vi "Test API Creates Report If No Tests Are Run.vi"(8 "error in (no error)":errorcluster, 11 "API Test in":refnum<class "API Test.lvclass">) -> (0 "error out":errorcluster, 3 "API Test out":refnum<class "API Test.lvclass">)   [LabVIEW 2020, in "LUnit Tests.lvlib" / "API Test.lvclass"]
uses:
  API Test.lvclass
  C:/Program Files (x86)/National Instruments/LabVIEW 2020/vi.lib/Astemes/LUnit/Test Case.lvclass
  <vilib>/Astemes/LUnit/Test Case.lvclass/Test Case.ctl
  <vilib>/Astemes/LUnit/Palette/Fail.vi
  <vilib>/Astemes/LUnit/Palette/Pass.vi
  <vilib>/Astemes/LUnit/Set Assertion Type.vi
  <vilib>/Astemes/LUnit/Add test result.vi
  <vilib>/Astemes/LUnit/LUnit Record Assertion Result.vi
  <vilib>/Astemes/LUnit/LUnit Aggregate Assertion Results.vi
  <vilib>/Astemes/LUnit/Method Result/LUnit Merge Status.vi
  <vilib>/Astemes/LUnit/LUnit Concatenate result strings.vi
  API Test.lvclass/API Test.ctl
  source/Framework/Execution API/Execution API.lvclass
  <vilib>/Astemes/LUnit/Test Case.lvclass
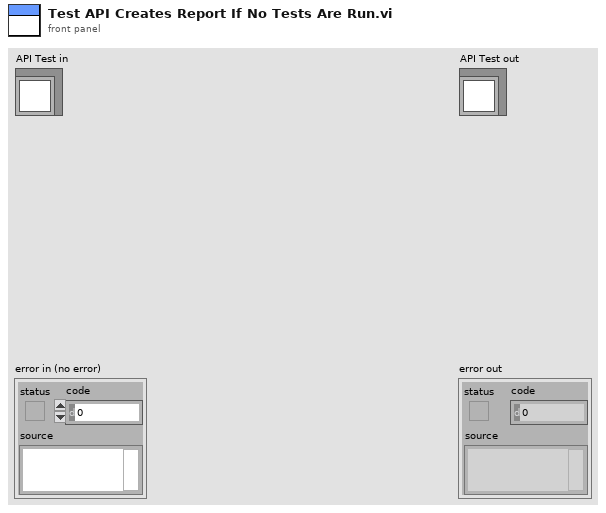
[diagram p1: front panel]
types:
  T1 = cluster{"Result Events":refnum<event-registration>, "Event Registration Refnum":refnum<event-registration>}
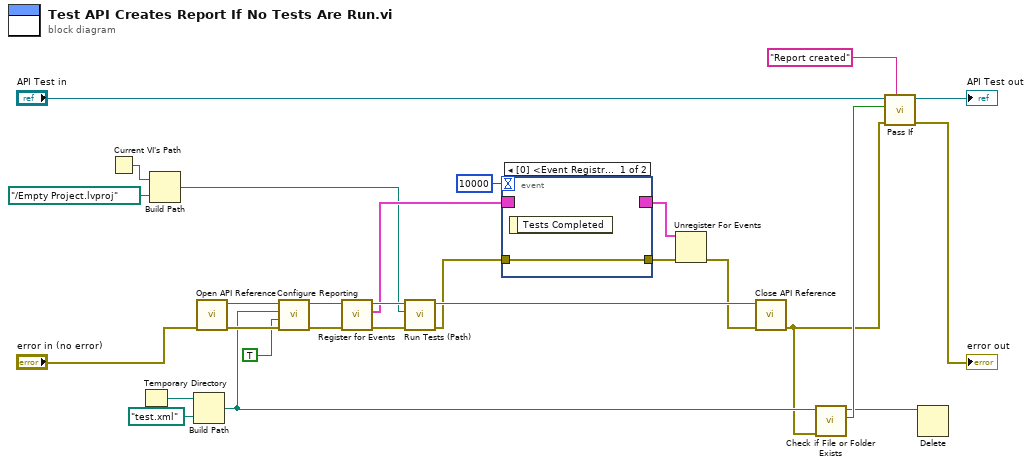
[diagram p0: block diagram]
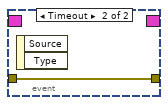
[diagram p2: hidden frame]
diagram:
  n1 = Current VI's Path() -> (path=w3:path)
  n2 = Temporary Directory() -> (w19:path)
  n3 = Build Path(base path=w3, name or relative path=path "../Empty Project.lvproj") -> (appended path=w1:path)
  n4 = Build Path(base path=w19, name or relative path=path "test.xml") -> (appended path=w16:path)
  n5 = call "Open API Reference.vi"("error in (no error)"="error in (no error)") -> ("error out"=w21:errorcluster, "Execution API out"=w22:refnum<class "Execution API.lvclass">)  [unwired: 9 in]
  n6 = call "Configure Reporting.vi"("error in (no error)"=w21, "Autogenerate?"=TRUE, "Path"=w16, "Execution API In"=w22) -> ("error out"=w20:errorcluster, "Execution API Out"=w6:refnum<class "Execution API.lvclass">)  [unwired: 6 in]
  n7 = call "Register for Events.vi"("error in (no error)"=w20, "Execution API in"=w6) -> ("error out"=w7:errorcluster, "Event Registrations"=w4:T1, "Execution API out"=w5:refnum<class "Execution API.lvclass">)  [unwired: 7 in]
  n8 = call "Run Tests (Path).vi"("error in (no error)"=w7, "Project or Class Path"=w1, "Execution API In"=w5) -> ("error out"=w27:errorcluster, "Execution API Out"=w28:refnum<class "Execution API.lvclass">)  [unwired: 7 in]
  n9 = event shown="[0] <Event Registration Refnum.Test Completed>: User Event" {
    selector: w4 -> [_ _]
    dyn-events: [_ _] -> w25
    timeout: 10000 -> [_ _]
    tunnel: w27 -> [w29 w30]
    tunnel: [w29 w30] -> w24
    event User Event {
      n10 = event-data() -> ()  [unwired: 1 in, 1 out]
    }
    event Timeout {
      n11 = event-data() -> ()  [unwired: 1 in, 2 out]
    }
  }
  n12 = Unregister For Events(event registration refnum=w25, error in=w24) -> (error out=w26:errorcluster)
  n13 = call "Close API Reference.vi"("error in (no error)"=w26, "Execution API in"=w28) -> ("error out"=w10:errorcluster)  [unwired: 9 in]
  n14 = call <vilib>:"Check if File or Folder Exists.vi"("error in (no error)"=w10, "path"=w16) -> ("file or folder exists?"=w13:bool, "dup path"=w12:path)  [unwired: 7 in, 1 out]
  n15 = call <vilib>:"Pass If.vi"("Description"="Report created", "error in (no error)"=w10, "Pass?"=w13, "LUnit Test Case In"="API Test in") -> ("error out"=→"error out":errorcluster, "LUnit Test Case Out"=→"API Test out":refnum<class "API Test.lvclass">)  [unwired: 6 in]
  n16 = Delete(path (use dialog)=w12) -> ()  [unwired: 4 in, 3 out]
